vi "Close.vi"(8 "error in (no error)":errorcluster, 11 "1553 Board in":refnum<class "1553 Session.lvclass">) -> (0 "error out":errorcluster)   [LabVIEW 2020, in "BCI-1553 API.lvlib" / "1553 Session.lvclass"]
doc: "Closes all the references and sessions opened by the 1553 Session. It is recommended to call the 'Stop' method before calling this if a 1553 Session was started."
uses:
  1553 Session.lvclass
  1553 Session.lvclass/1553 Session.ctl
  1553 Component/1553 Component.lvclass
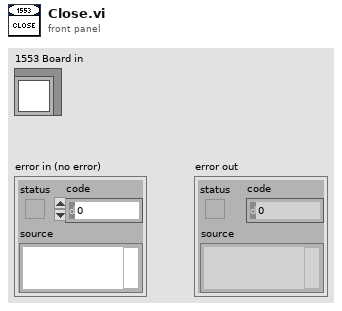
[diagram p1: front panel]
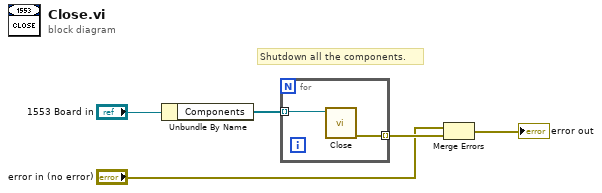
[diagram p0: block diagram]
diagram:
  # "Shutdown all the components."
  n1 = Unbundle By Name("1553 Board in") -> ("Components"=w3:refnum<class "1553 Component.lvclass">[])
  n2 = for {
    tunnel: [w7] -> w5 mode=indexing
    tunnel: w3 -> [w6] mode=indexing
    n3 = call-dynamic "Close.vi"("1553 Component in"=w6) -> ("error out"=w7:errorcluster)  [unwired: 10 in]
  }
  n4 = Merge Errors("error in (no error)", w5) -> (→"error out":errorcluster)
